vi "LabVIEW Coordinates to Picture Coordinates.vi"(8 "entrée d'erreur":errorcluster, 10 "RéfCmde":refnum<vi>, 11 "Coordonnées LabVIEW":cluster{"Horizontale":i32, "Verticale":i32}) -> (0 "sortie d'erreur":errorcluster, 3 "Coordonnées de la commande image":cluster{"Horizontale":i32, "Verticale":i32})   [LabVIEW 2009]
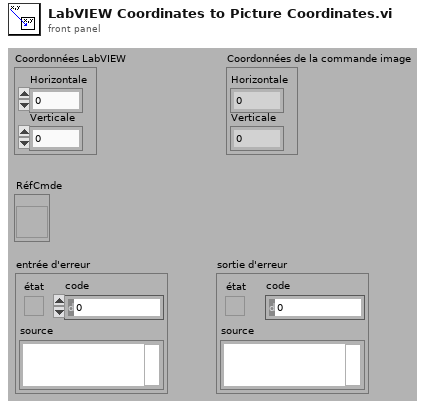
[diagram p1: front panel]
types:
  T1 = typedef "LVBoundsTypeDef.ctl" = cluster{"Width":u32, "Height":u32}
  T2 = typedef "LVPositionTypeDef.ctl" = cluster{"Left":i32, "Top":i32}
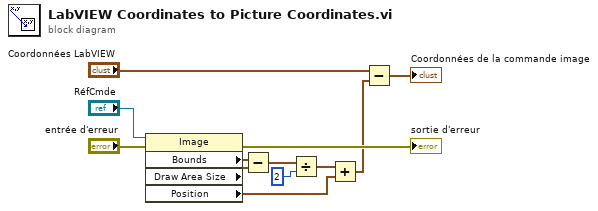
[diagram p0: block diagram]
diagram:
  n1 = property on="Nœud de propriété" class="Image"(reference="RéfCmde", error in="entrée d'erreur") -> (error out=→"sortie d'erreur":errorcluster, "Bounds"=w3:T1, "Draw Area Size"=w4:T1, "Position"=w8:T2)  [unwired: 1 out]
  n2 = Subtract ("Soustraire")(x=w3, y=w4) -> (x-y=w6:T1)
  n3 = Divide ("Diviser")(x=w6, y=2) -> (x/y=w7:cluster{"Width":dbl, "Height":dbl})
  n4 = Add ("Additionner")(x=w7, y=w8) -> (x+y=w10:cluster{dbl, dbl})
  n5 = Subtract ("Soustraire")(x="Coordonnées LabVIEW", y=w10) -> (x-y=→"Coordonnées de la commande image":cluster{dbl, dbl})
